vi "ti2_open.vi"(8 "error in (no error)":errorcluster) -> (0 "error out":errorcluster)   [LabVIEW 2018, in "ti2lv.lvlib"]
uses:
  ti2lv.lvlib
  ti2wrap/x64/Release/ti2wrap.dll
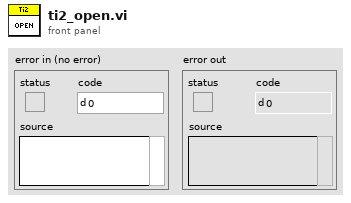
[diagram p1: front panel]
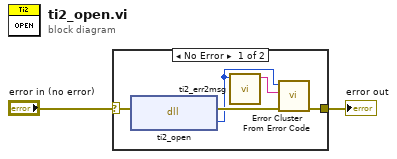
[diagram p0: block diagram]
diagram:
  n1 = case shown="No Error" "error in (no error)" {
    selector: "error in (no error)" -> [w6 w8]
    tunnel: [w7 w8] -> w1
    frame No Error {
      n2 = dll-call lib="C:/LVFAST/Flash Gordon v0.6.1b/Hardware/Ti2/ti2wrap/x64/Release/ti2wrap.dll" fn="ti2_open"(error in=w6) -> (error out=w5:errorcluster, "return type"=w4:i32)  [unwired: 2 in, 1 out]
      n3 = call "ti2_err2msg.vi"("Error Code"=w4) -> ("Error Message"=w3:string)  [unwired: 10 in]
      n4 = call <vilib>:"Error Cluster From Error Code.vi"("error in (no error)"=w5, "error message (\"\")"=w3, "error code (0)"=w4) -> ("error out"=w7:errorcluster)  [unwired: 6 in]
    }
    frame Error {
    }
  }
  "error out" <- w1
